vi "LVClass_CameraSet Read CameraSet.vi"(8 "error in (no error)":errorcluster, 11 "CameraSet in":refnum<class "CameraSet.lvclass">) -> (0 "error out":errorcluster, 2 "camera":T1, 3 "CameraSet out":refnum<class "CameraSet.lvclass">)   [LabVIEW 2020, in "CameraSet.lvclass"]
uses:
  CameraSet.lvclass
  CameraSet.ctl
  CameraSet.lvclass/CameraSet.ctl
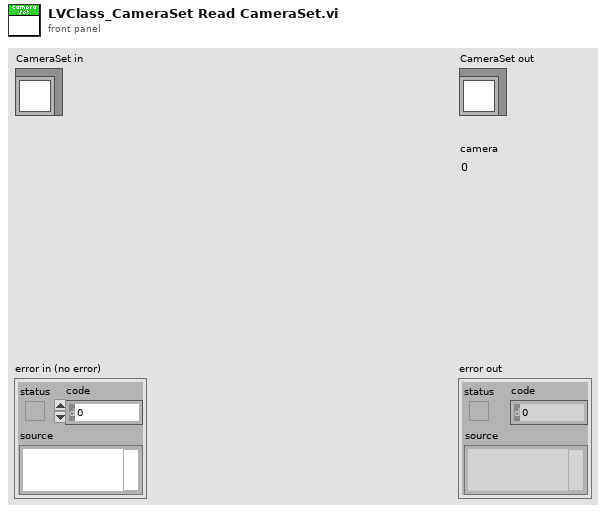
[diagram p1: front panel]
types:
  T1 = typedef "CameraSet.ctl" = i32
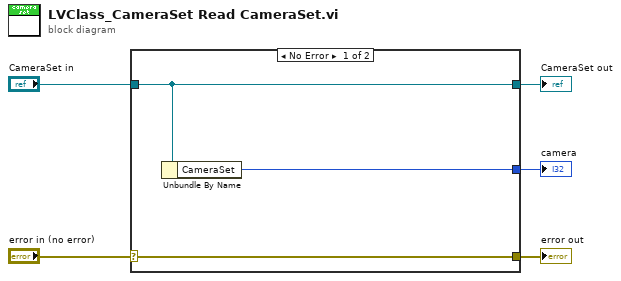
[diagram p0: block diagram]
diagram:
  n1 = case shown="No Error" "error in (no error)" {
    selector: "error in (no error)" -> [w8 w9]
    tunnel: [w8 w9] -> w4
    tunnel: [w7 w10] -> w2
    tunnel: "CameraSet in" -> [w7 w10]
    tunnel: [w6 _] -> w1
    frame No Error {
      n2 = Unbundle By Name(w7) -> ("CameraSet"=w6:T1)
    }
    frame Error {
    }
  }
  "error out" <- w4
  "CameraSet out" <- w2
  "camera" <- w1
